vi "filter_control_key_down.vi"(8 "error in (no error)":errorcluster, 10 "Ctl Refnum":refnum<vi>, 11 "IControlShortcutMenu In":refnum<class "IControlKeyDownFilter.lvclass">) -> (0 "error out":errorcluster, 2 "Discarded?":bool, 3 "IControlShortcutMenu Out":refnum<class "IControlKeyDownFilter.lvclass">)   [LabVIEW 2015, in "ActorEvents.lvlib" / "IControlKeyDownFilter.lvclass"]
uses:
  IControlKeyDownFilter.lvclass
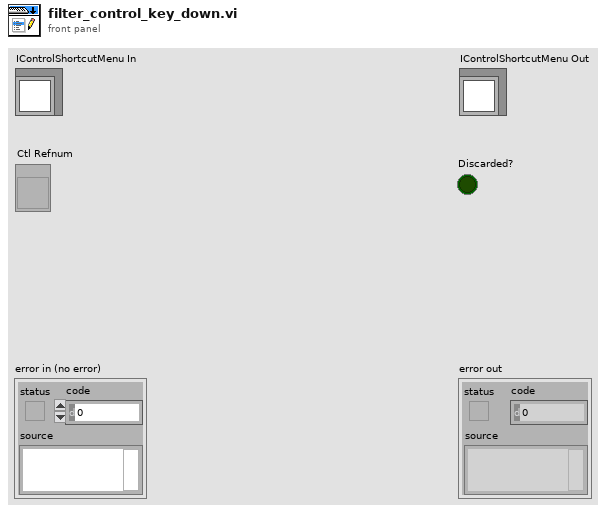
[diagram p1: front panel]
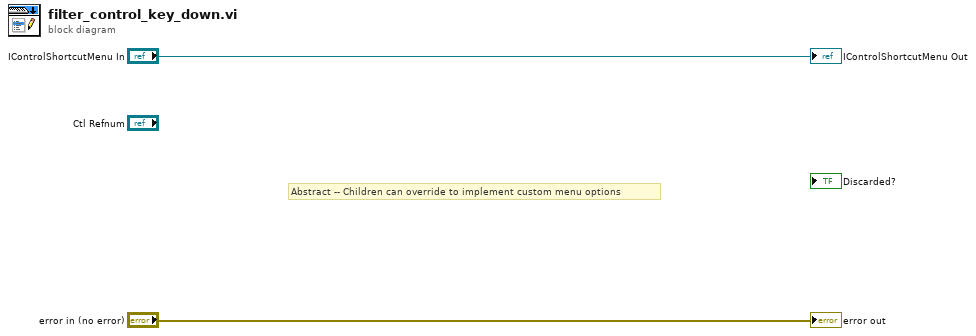
[diagram p0: block diagram]
diagram:
  # "Abstract -- Children can override to implement custom menu options"
  "error out" <- "error in (no error)"
  "IControlShortcutMenu Out" <- "IControlShortcutMenu In"
